vi "Display Attendance Result(UI).vi"(8 "error in (no error)":errorcluster, 9 "Name(\"\")":string, 10 "Department(\"\")":string, 11 "CalAttendance in":refnum<class "CalAttendance.lvclass">) -> (0 "error out":errorcluster, 1 "NumOfAttendance":T1, 2 "Res_Attendance":cluster{"BackGround":u32, "Reason":string}[][](array[cluster]), 3 "CalAttendance out":refnum<class "CalAttendance.lvclass">)   [LabVIEW 2015, in "Admin_Actor.lvlib" / "CalAttendance.lvclass"]
uses:
  CalAttendance.lvclass
  Type Definitions/NumOfAttendace.ctl
  Models/Attendance Record/AttendRecord.lvclass
  CalAttendance.lvclass/CalAttendance.ctl
  Models/Attendance Record/AttendRecord.lvclass/AttendRecord.ctl
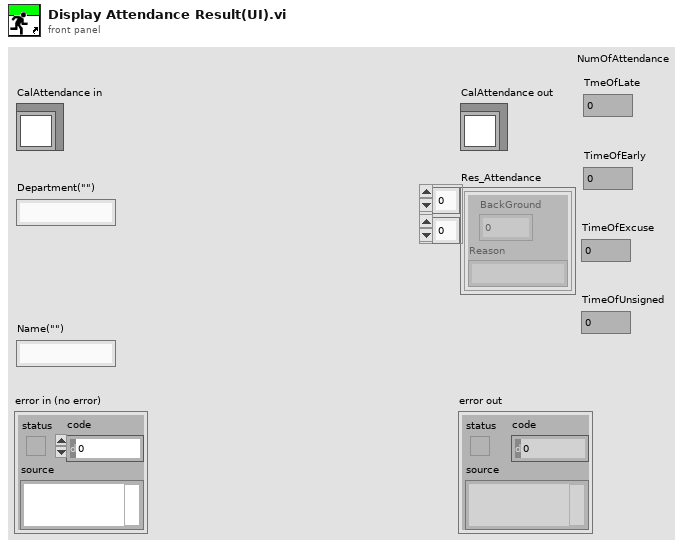
[diagram p1: front panel]
types:
  T1 = typedef "Admin_Actor.lvlib/CalAttendance.lvclass/NumOfAttendace.ctl" = cluster{"TmeOfLate":i32, "TimeOfEarly":i32, "TimeOfExcuse":i32, "TimeOfUnsigned":i32}
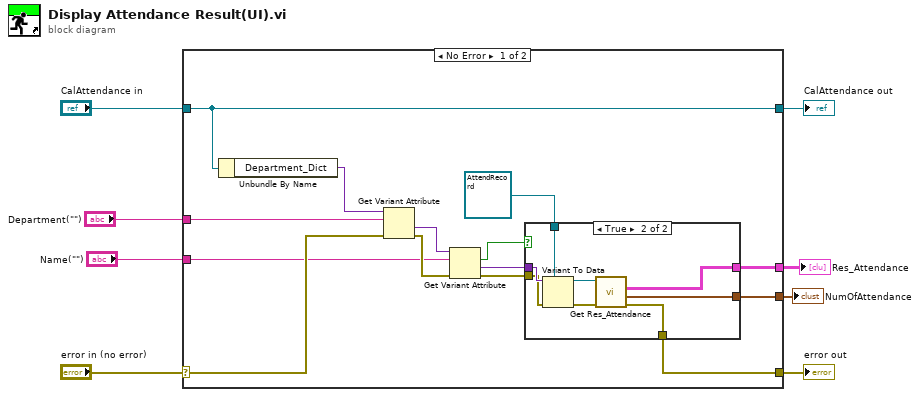
[diagram p0: block diagram]
diagram:
  n1 = case shown="No Error" "error in (no error)" {
    selector: "error in (no error)" -> [w19 w33]
    tunnel: [w15 w33] -> w7
    tunnel: [w22 w32] -> w5
    tunnel: "CalAttendance in" -> [w22 w32]
    tunnel: "Name(\"\")" -> [w9 _]
    tunnel: "Department(\"\")" -> [w10 _]
    tunnel: [w14 _] -> w2
    tunnel: [w13 _] -> w1
    frame No Error {
      n2 = Unbundle By Name(w22) -> ("Department_Dict"=w21:variant)
      n3 = Get Variant Attribute(Variant=w21, name=w10, error in=w19) -> (value=w20:variant, error out=w18:errorcluster)  [unwired: 1 in, 2 out]
      n4 = Get Variant Attribute(Variant=w20, name=w9, error in=w18) -> (found=w11:bool, value=w17:variant, error out=w16:errorcluster)  [unwired: 1 in, 1 out]
      n5 = case shown="True" w11 {
        tunnel: w17 -> [_ w31]
        tunnel: w16 -> [w23 w30]
        tunnel: [w23 w27] -> w15
        tunnel: [_ w26] -> w14
        tunnel: [_ w25] -> w13
        tunnel: refnum<class "AttendRecord.lvclass"> refnum ("AttendRecord.lvclass") -> [_ w24]
        frame False {
        }
        frame True {
          n6 = Variant To Data(error in=w30, type=w24, Variant=w31) -> (data=w29:refnum<class "AttendRecord.lvclass">, error out=w28:errorcluster)
          n7 = call "Get Res_Attendance.vi"("error in (no error)"=w28, "AttendRecord in"=w29) -> ("error out"=w27:errorcluster, "NumOfAttendance"=w25:T1, "Res_Attendance"=w26:cluster{"BackGround":u32, "Reason":string}[][])  [unwired: 6 in, 1 out]
        }
      }
    }
    frame Error {
    }
  }
  "error out" <- w7
  "CalAttendance out" <- w5
  "Res_Attendance" <- w2
  "NumOfAttendance" <- w1
